vi "Math-Bernoulli Trial.vi"(0 "samples":i32=1, 5 "U":dbl, 7 "X":dbl[](array[numeric]), 9 "PofX":dbl[](array[numeric]), 11 "interpolate":bool) -> (4 "Array":dbl[](array[numeric]), 8 "Prob":dbl)   [LabVIEW 2020]
uses:
  LinSpace (x0-dx-npts).vi
  21bb566b-05c2-44e4-af54-d93bd0e4d667.vi
  e49c2c3f-b004-4adc-9947-8f4e65aa1f3a.vi
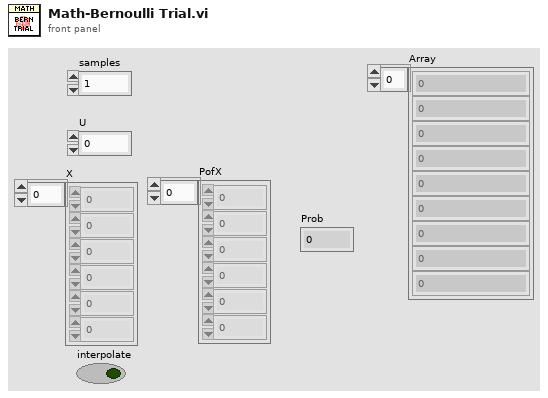
[diagram p1: front panel]
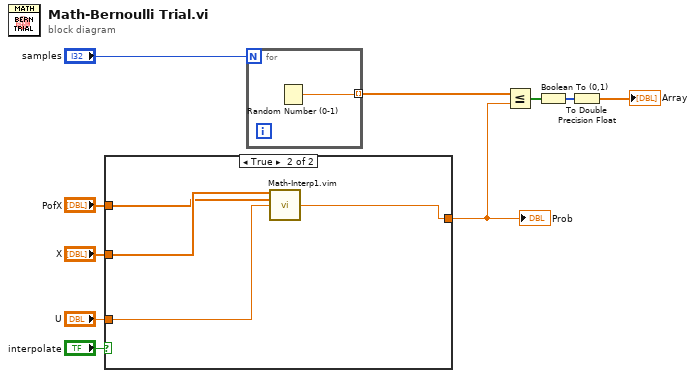
[diagram p0: block diagram]
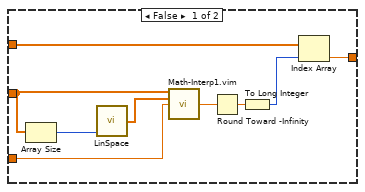
[diagram p2: hidden frame]
diagram:
  n1 = case shown="True" "interpolate" {
    tunnel: "X" -> [w19 w23]
    tunnel: "U" -> [w16 w21]
    tunnel: "PofX" -> [w13 w22]
    tunnel: [w11 w20] -> w5
    frame False {
      n2 = Array Size(array=w19) -> (size(s)=w18:i32)
      n3 = call-poly "LinSpace.vi"("npts"=w18) -> ("Array"=w17:dbl[])  [unwired: 3 in, 1 out]
      n4 = call "Math-Interp1.vim"("X"=w19, "Y"=w17, "U"=w16) -> ("V"=w15:dbl)  [unwired: 12 in]
      n5 = Round Toward -Infinity(1:w15) -> (0:w14:dbl)
      n6 = To Long Integer(number=w14) -> (32bit integer=w12:i32)
      n7 = Index Array(array=w13, index=w12) -> (element=w11:dbl)
    }
    frame True {
      n8 = call "Math-Interp1.vim"("X"=w23, "Y"=w22, "U"=w21) -> ("V"=w20:dbl)  [unwired: 12 in]
    }
  }
  "Prob" <- w5
  n9 = for {
    N: "samples" -> [_]
    tunnel: [w24] -> w6 mode=indexing
    n10 = Random Number (0-1)() -> (number: 0 to 1=w24:dbl)
  }
  n11 = Less Or Equal?(x=w6, y=w5) -> (x <= y?=w4:bool[])
  n12 = Boolean To (0,1)(Boolean=w4) -> (0, 1=w3:i16[])
  n13 = To Double Precision Float(number=w3) -> (double precision float=→"Array":dbl[])
